vi "SendValue2000.vi"(0 "ip":string, 1 "command":string, 2 "Stringvalue":string, 4 "Boolean":bool, 5 "value":dbl, 6 "connection ID":refnum<k16>, 9 "Send Bool":bool) -> ()   [LabVIEW 2017]
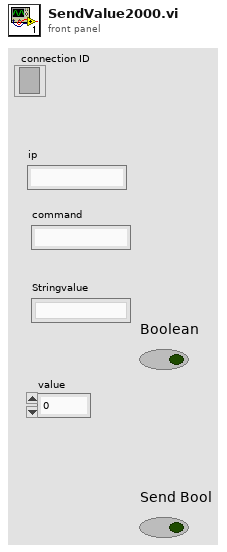
[diagram p1: front panel]
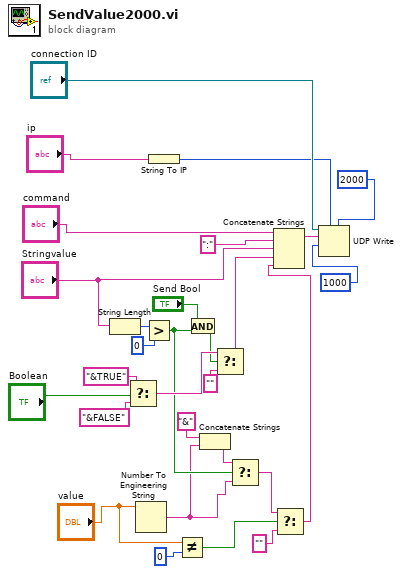
[diagram p0: block diagram]
diagram:
  n1 = String Length(string="Stringvalue") -> (length=w13:i32)
  n2 = Select(t="&TRUE", s="Boolean", f="&FALSE") -> (s? t:f=w11:string)
  n3 = Number To Engineering String(4:"value") -> (0:w3:string)  [unwired: 3 in]
  n4 = Greater?(x=w13, y=0) -> (0:w5:bool)
  n5 = String To IP(1:"ip") -> (0:w26:u32)
  n6 = Not Equal?(x="value", y=0) -> (x != y?=w18:bool)
  n7 = And(x="Send Bool", y=w5) -> (x .and. y?=w7:bool)
  n8 = Concatenate Strings("&", w3) -> (w4:string)
  n9 = Select(t=w11, s=w7, f="") -> (s? t:f=w9:string)
  n10 = Select(t=w4, s=w5, f=w3) -> (s? t:f=w1:string)
  n11 = Select(t=w1, s=w18, f="") -> (s? t:f=w6:string)
  n12 = Concatenate Strings("command", ":", "Stringvalue", w9, w6) -> (w24:string)
  n13 = UDP Write(address=w26, port or service name=2000, connection ID="connection ID", data in=w24, 9:1000) -> ()  [unwired: 1 in, 2 out]
